vi "fetch.vi"(8 "error in (no error)":errorcluster, 10 "key chain":string[](array[string]), 11 "Map in":refnum<class "Map.lvclass">) -> (0 "error out":errorcluster, 1 "submap":refnum<class "Map.lvclass">, 2 "value":variant, 3 "Map out":refnum<class "Map.lvclass">, 4 "is it a submap?":bool, 5 "found?":bool)   [LabVIEW 2010, in "Map.lvclass"]
doc: "Returns a value. The position is specified by the key array. \nFor a nested map, the key array contains all keys from root down to the desired position. If the key array refers to non-existing intermediary nodes, these are created on the fly. \nFor a non-nested map, simply provide an array with a single key value."
uses:
  Map.lvclass
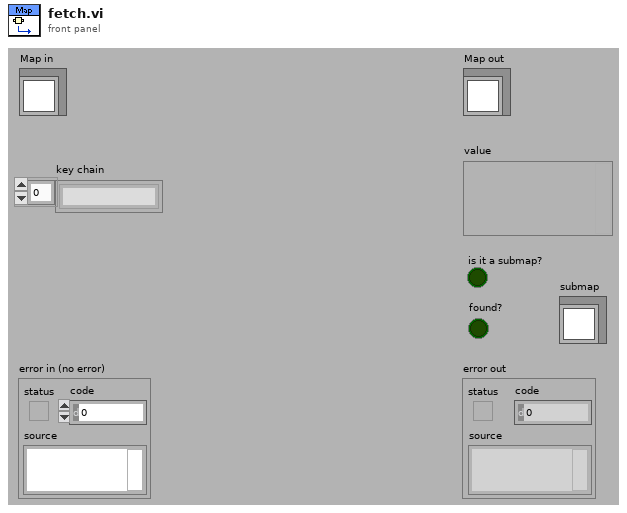
[diagram p1: front panel]
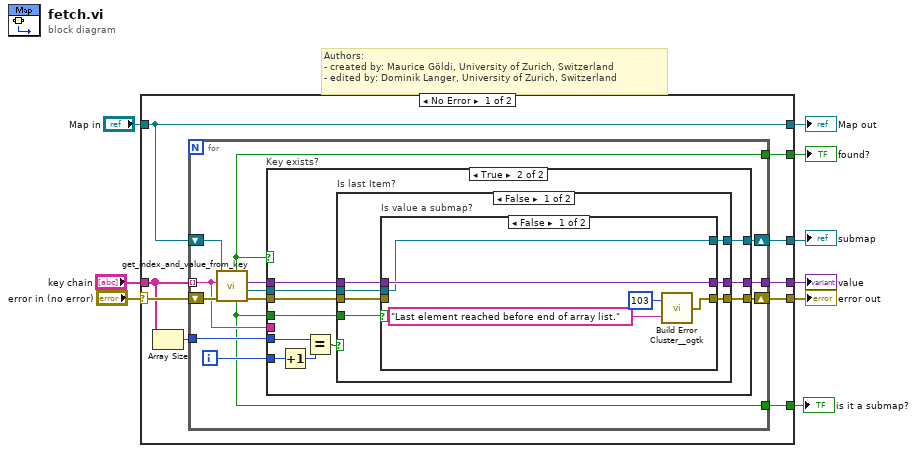
[diagram p0: block diagram]
diagram:
  # "Authors: \n- created by: Maurice Göldi, University of Zurich, Switzerland\n- edited by: Dominik Langer, University of Zurich, Switzerland"
  n1 = case shown="No Error" "error in (no error)" {
    selector: "error in (no error)" -> [w18 w65]
    tunnel: [w17 w65] -> w8
    tunnel: [w16 w64] -> w6
    tunnel: "Map in" -> [w16 w64]
    tunnel: "key chain" -> [w14 _]
    tunnel: [w15 _] -> w4
    tunnel: [w12 _] -> w3
    tunnel: [w11 _] -> w2
    tunnel: [w10 _] -> w1
    frame No Error {
      n2 = Array Size(array=w14) -> (size(s)=w13:i32)
      n3 = for {
        shift-right: [w22] -> w17
        shift-left: w18 -> [w29]
        tunnel: w14 -> [w21] mode=indexing
        shift-right: [w31] -> w11
        shift-left: w16 -> [w27]
        tunnel: [w30] -> w15
        tunnel: w13 -> [w23]
        tunnel: [w20] -> w12
        tunnel: [w19] -> w10
        i -> [w24]
        n4 = call "get_index_and_value_from_key.vi"("error in (no error)"=w29, "key"=w21, "Map.lvclass in"=w27) -> ("error out"=w28:errorcluster, "submap"=w25:refnum<class "Map.lvclass">, "value"=w26:variant, "submap?"=w20:bool, "key exists?"=w19:bool)  [unwired: 4 out]
        n5 = case "Key exists?" shown="True" w19 {
          tunnel: w28 -> [w32 w42]
          tunnel: [w33 w37] -> w31
          tunnel: [w34 w41] -> w30
          tunnel: w26 -> [w34 w40]
          tunnel: w25 -> [w33 w38]
          tunnel: w20 -> [_ w43]
          tunnel: w24 -> [_ w36]
          tunnel: w23 -> [_ w45]
          tunnel: [w32 w39] -> w22
          tunnel: w21 -> [_ _]
          frame False {
          }
          frame True {
            n6 = Increment(x=w36) -> (x+1=w35:i32)
            n7 = Equal?(x=w45, y=w35) -> (x = y?=w44:bool)
            n8 = case "Is last Item?" shown="False" w44 {
              tunnel: w43 -> [w50 _]
              tunnel: w42 -> [w49 w62]
              tunnel: [w51 w63] -> w41
              tunnel: w40 -> [w52 w63]
              tunnel: [w48 w62] -> w39
              tunnel: w38 -> [w47 w61]
              tunnel: [w46 w61] -> w37
              frame False {
                n9 = case "Is value a submap?" shown="False" w50 {
                  tunnel: w52 -> [w57 w60]
                  tunnel: [w57 w60] -> w51
                  tunnel: w49 -> [_ w59]
                  tunnel: [w53 w59] -> w48
                  tunnel: w47 -> [w56 w58]
                  tunnel: [w56 w58] -> w46
                  frame False {
                    n10 = call <userlib>:"Build Error Cluster__ogtk.vi"("String to Prepend to source (\"\")"="Last element reached before end of array list." ("string"), "code"=103) -> ("error out"=w53:errorcluster)
                  }
                  frame True {
                  }
                }
              }
              frame True {
              }
            }
          }
        }
      }
    }
    frame Error {
    }
  }
  "error out" <- w8
  "Map out" <- w6
  "value" <- w4
  "is it a submap?" <- w3
  "submap" <- w2
  "found?" <- w1
